vi "TB3000_amplitude_query.vi"(8 "Error In":errorcluster, 11 "VISA resource name in":refnum<visa-resource-name>) -> (0 "Error Out":errorcluster, 2 "amplitude (%)":dbl, 3 "VISA resource name out":refnum<visa-resource-name>)   [LabVIEW 2021]
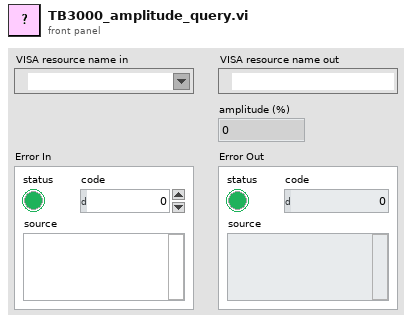
[diagram p1: front panel]
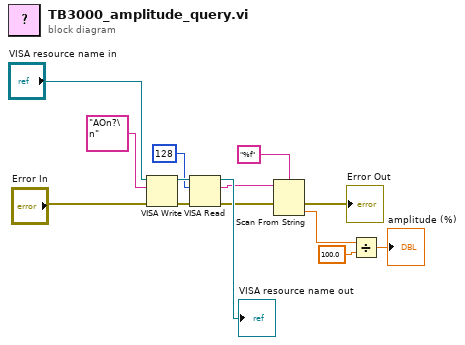
[diagram p0: block diagram]
diagram:
  n1 = VISA Write(VISA resource name="VISA resource name in", write buffer="AOn?\n", error in (no error)="Error In") -> (VISA resource name out=w14:refnum<visa-resource-name>, error out=w13:errorcluster)  [unwired: 1 out]
  n2 = VISA Read(VISA resource name=w14, byte count=u32 128, error in (no error)=w13) -> (VISA resource name out=→"VISA resource name out":refnum<visa-resource-name>, read buffer=w8:string, error out=w7:errorcluster)  [unwired: 1 out]
  n3 = Scan From String(format string="%f", input string=w8, error in=w7) -> (error out=→"Error Out":errorcluster, output 1=w4:dbl)  [unwired: 2 in, 2 out]
  n4 = Divide(x=w4, y=100.0) -> (x/y=→"amplitude (%)":dbl)
